vi "Sample Panel2.vi"(8 "error in (no error)":errorcluster, 9 "Left Or Right":string, 10 "Measure_No":i64, 11 "connection reference":T1) -> (0 "error out":errorcluster)   [LabVIEW 2015, in "Sample.lvlib"]
uses:
  Sample.lvlib
  <vilib>/addons/database/Connection.llb/Conn ObjectReference.ctl
  <vilib>/userdefined/High Color/IMAQdx.ctl
  Sub VIs/CCD/CCD.lvlib
  Sub VIs/DAQ/DAQ.lvlib
  <vilib>/vision/driver/NI_Vision_Acquisition_Software.lvlib
  Sub VIs/Digital Signal Processing/Digital Signal Processing.lvlib
  Sub VIs/Utility VIs/Utility VIs.lvlib
  Sub VIs/Database Processing/Database Processing.lvlib
  <vilib>/addons/database/NI_Database_API.lvlib
panel:
  in  "x":bool
  out "Asan Signal":dbl[](graph)
  out "CH1":dbl[](array[numeric])
  in  "停止":bool
  out "CCD Image":T2(plugin-control)
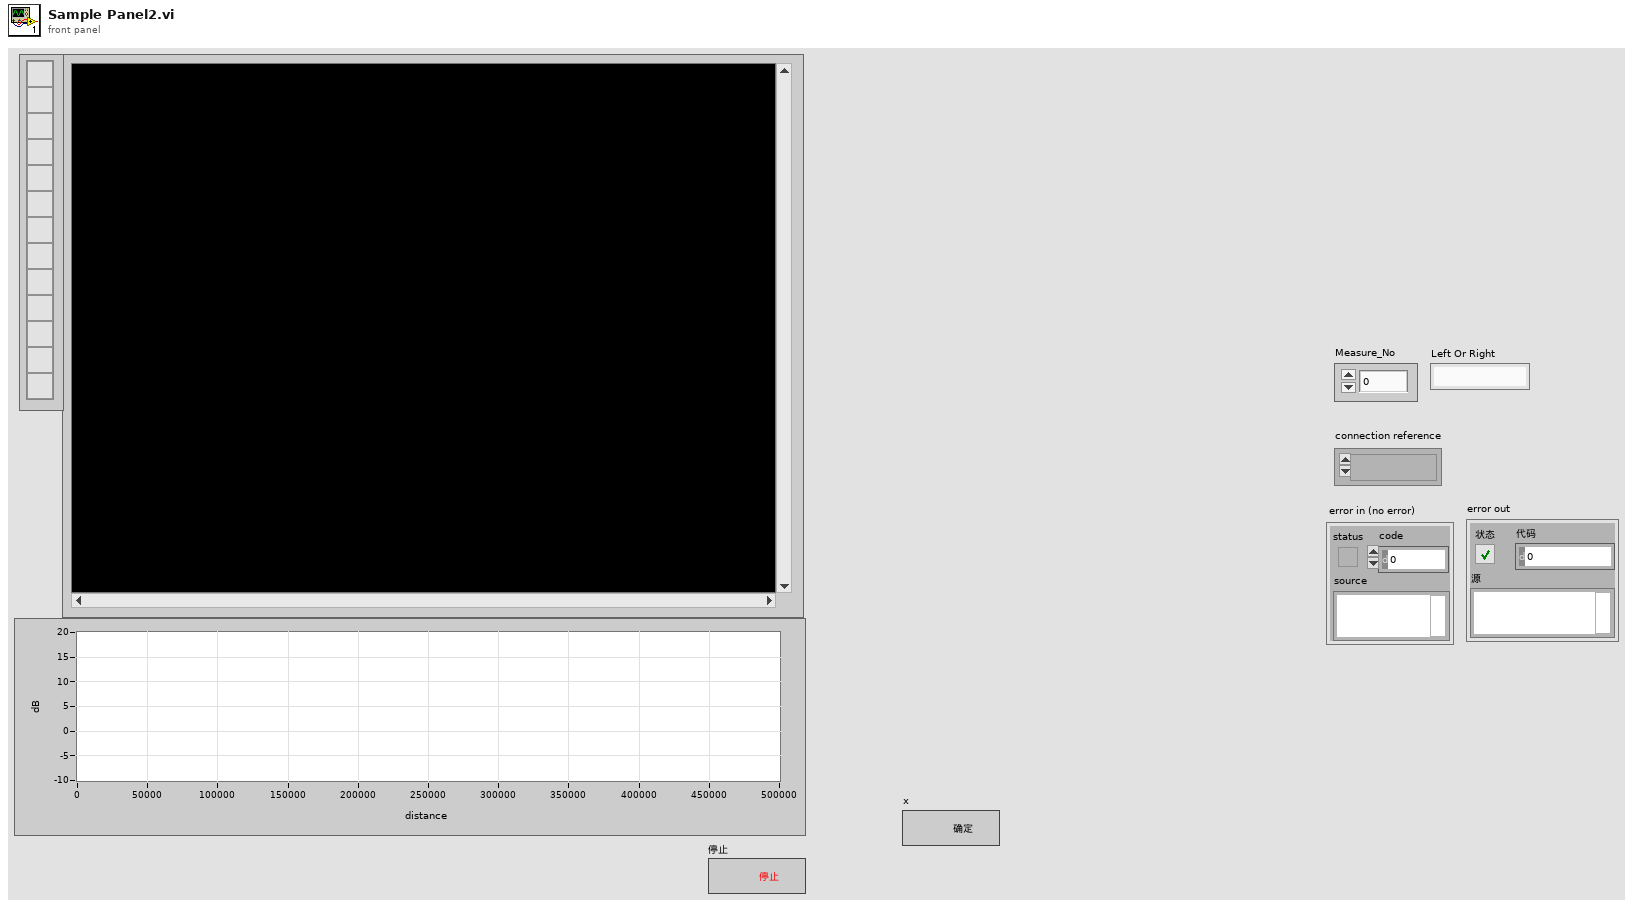
[diagram p1: front panel]
types:
  T1 = typedef "NI_Database_API.lvlib/Conn ObjectReference.ctl" = refnum<k1>
  T2 = typedef "IMAQ Image.ctl" = refnum<image>
  T3 = typedef "IMAQdx.ctl" = refnum<k21>
  T4 = typedef "Database Processing.lvlib/Biometry Attribute.ctl" = cluster{"Measure_ID":i64, "Measure_No":i64, "Ordinal":i64, "L_Or_R":string}
  T5 = typedef "DAQ.lvlib/DAQ Configuration.ctl" = cluster{"hDevice":i32, "DevNum":u8, "Configuration Parameter":i32[], "READ_MAX_LEN":i32, "DO":bool[]}
  T6 = typedef "Digital Signal Processing.lvlib/DSP Configuration.ctl" = cluster{"Sampling Frequency":dbl, "filter type":T7, "RF Filter Low Frequency":dbl, "RF Filter High Frequency":dbl, "RF Filter Taps":i32, "window":T8, "RF window parameter":dbl, "filter type 2":T7, "Demodulated Filter Low Frequency":dbl, "Demodulated Filter HighFrequency":dbl, "Demodulated Filter Order":i32, "SPAN":i32, "Logarithmic Base":dbl, "Noise path":string, "Work position parameter":i32[]}
  T7 = typedef "NI_AALBase.lvlib/Filter Passband Type.ctl" = enum32{"Lowpass", "Highpass", "Bandpass", "Bandstop"}
  T8 = typedef "NI_AALPro.lvlib/windowTd.ctl" = u32
  T9 = typedef "Digital Signal Processing.lvlib/DSP Parameter.ctl" = cluster{"RF":cluster{"filter structure":enum32{"IIR 2nd Order", "IIR 4th Order"}, "Reverse Coefficients":dbl[], "Forward Coefficients":dbl[]}, "IIR Filter Cluster":cluster{"filter structure":enum32{"IIR 2nd Order", "IIR 4th Order"}, "Reverse Coefficients":dbl[], "Forward Coefficients":dbl[]}, "Noise Signal":dbl[], "SPAN":i32, "Logarithmic Base":dbl}
  T10 = cluster{"Measure_ID":i32, "Original Ascan Path":string, "Original IR Path":string, "Original WTW Path":string, "Processing Ascan Path":string, "Processing IR Path":string, "Processing WTW Path":string, "Processing K Path":string, "Processing A Path":string}
  T11 = cluster{"Measure_ID":i32, "Measure_No":i32, "Ordinal":i32, "Left Or Right":string}
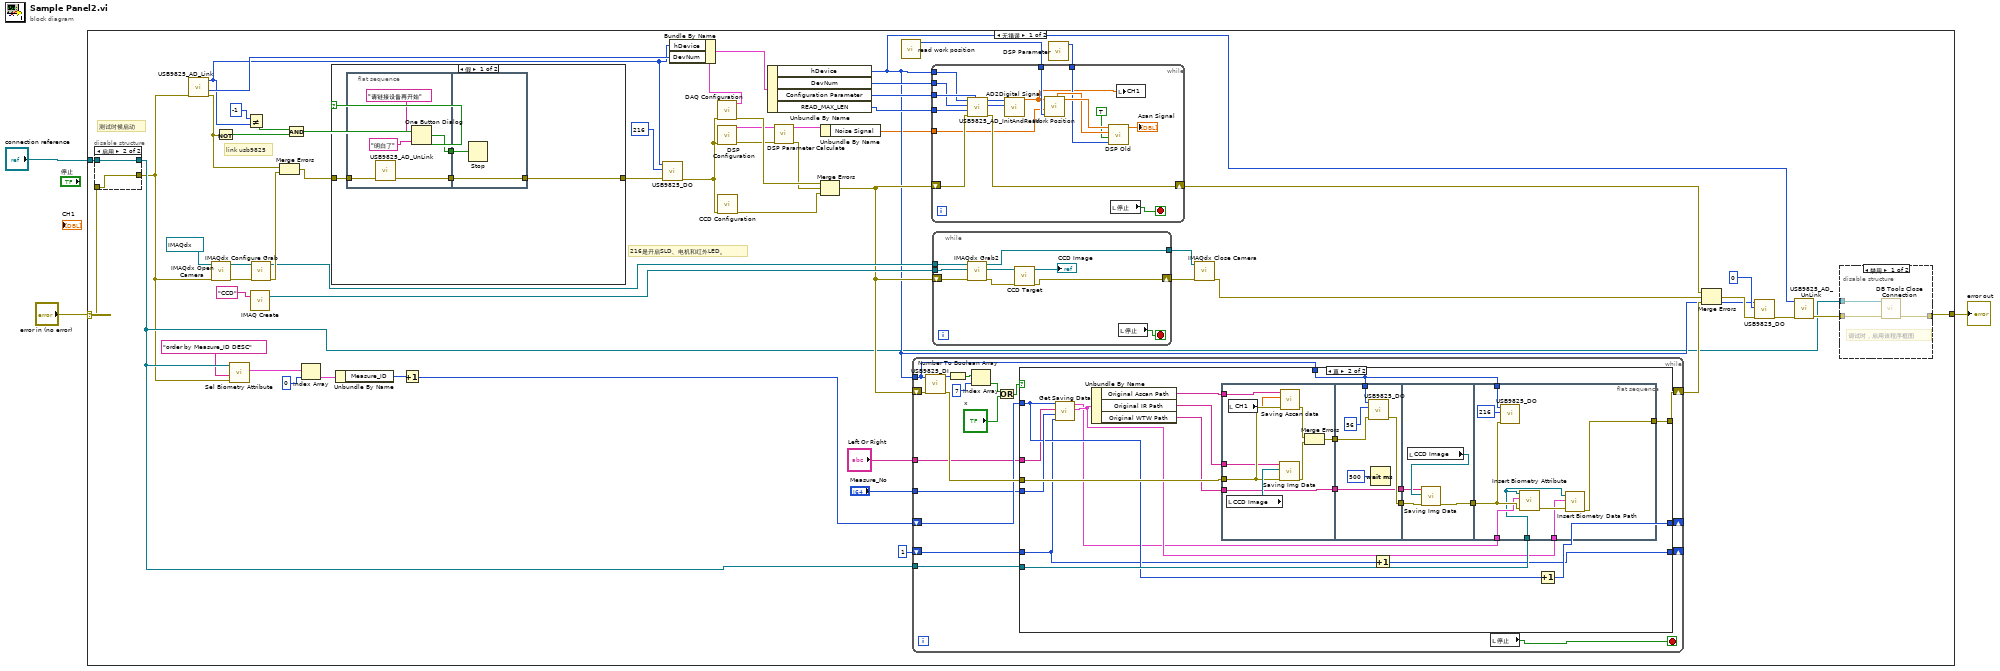
[diagram p0: block diagram]
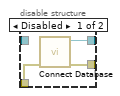
[diagram p3: hidden frame]
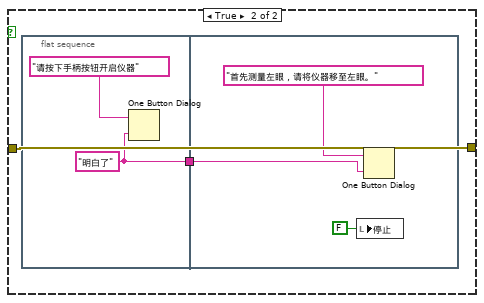
[diagram p5: hidden frame]
diagram:
  n1 = case shown="无错误" "error in (no error)" {
    selector: "error in (no error)" -> [w28 w182]
    tunnel: "connection reference" -> [w27 _]
    tunnel: [w20 w182] -> w1
    frame No Error {
      # "测试时候启动"
      # "216是开启SLD、电机和红外LED。"
      # "link usb9825"
      n2 = disable-structure shown="启用" {
        disable-tunnel: [w67 w68] -> w6
        disable-tunnel: w28 -> [w66 w68]
        disable-tunnel: [w65 w69] -> w8
        disable-tunnel: w27 -> [_ w69]
        frame Disabled {
          n3 = call "Connect Database.vi"("error in (no error)"=w66) -> ("error out"=w67:errorcluster, "connection reference"=w65:T1)  [unwired: 9 in]
        }
        frame Enabled {
        }
      }
      n4 = call "USB9825_AD_Link.vi"("Error In"=w6) -> ("Error Out"=w60:errorcluster, "DevNum"=w34:i32, "hDevice"=w33:i32)  [unwired: 7 in, 1 out]
      n5 = call <vilib>:"IMAQdx Open Camera.vi"("error in"=w6, "Session In"=T3 "cam0") -> ("error out"=w55:errorcluster, "Session Out"=w56:T3)  [unwired: 8 in]
      n6 = Not(x=w60) -> (.not. x?=w51:bool)
      n7 = call "Sel Biometry Attribute.vi"("error in (no error)"=w6, "condition"="order by Measure_ID DESC", "connection reference"=w8) -> ("Biometry Attribute"=w9:T4[])  [unwired: 7 in, 1 out]
      n8 = Not Equal?(x=-1, y=w33) -> (x != y?=w52:bool)
      n9 = call "IMAQ Create"("Image Name"="CCD") -> ("New Image"=w39:T2)  [unwired: 4 in, 1 out]
      n10 = call <vilib>:"IMAQdx Configure Grab.vi"("error in"=w55, "Session In"=w56) -> ("error out"=w53:errorcluster, "Session Out"=w40:T3)  [unwired: 8 in]
      n11 = Merge Errors(w60, w53) -> (w58:errorcluster)
      n12 = And(x=w52, y=w51) -> (x .and. y?=w50:bool)
      n13 = Index Array(array=w9, index=0 ("索引")) -> (element=w26:T4)
      n14 = case shown="假" w50 {
        tunnel: [w167 w175] -> w49
        tunnel: w58 -> [w166 w175]
        frame False {
          n15 = flat-sequence {
            tunnel: [w168] -> w165
            tunnel: w166 -> [w169]
            tunnel: [w170] -> w164
            tunnel: [w173] -> w167
            tunnel: w165 -> [w173]
            tunnel: w164 -> [w174]
            frame #0 {
              n16 = call "USB9825_AD_UnLink.vi"("Error In"=w169) -> ("Error Out"=w168:errorcluster)  [unwired: 10 in]
              n17 = One Button Dialog(message="请链接设备再开始" ("消息"), button name ("OK")="明白了" ("按钮名称（“确定”）")) -> (true=w170:bool)
            }
            frame #1 {
              n18 = Stop(stop? (T)=w174) -> ()
            }
          }
        }
        frame True {
          n19 = flat-sequence {
            tunnel: [w177] -> w176
            tunnel: w176 -> [w181]
            frame #0 {
              w177 = "明白了" ("按钮名称（“确定”）")
              n20 = One Button Dialog(message="请按下手柄按钮开启仪器" ("消息"), button name ("OK")=w177) -> ()  [unwired: 1 out]
            }
            frame #1 {
              n21 = local write "停止"(FALSE ("停止")) -> ()
              n22 = One Button Dialog(message="首先测量左眼，请将仪器移至左眼。" ("消息"), button name ("OK")=w181) -> ()  [unwired: 1 out]
            }
          }
        }
      }
      n23 = Unbundle By Name(w26) -> ("Measure_ID"=w24:i64)
      n24 = Increment(x=w24) -> (x+1=w23:i64)
      n25 = call "USB9825_DO.vi"("Error In"=w49, "pDO"=u8 216, "hDevice"=w33) -> ("Error Out"=w38:errorcluster)  [unwired: 8 in]
      n26 = call "DAQ Configuration.vi"("error in (no error)"=w38) -> ("error out"=w47:errorcluster, "parameter output"=w36:T5)  [unwired: 9 in]
      n27 = Bundle By Name(cluster=w36, "hDevice"=w33, "DevNum"=w34) -> (w35:T5)
      n28 = call "DSP Configuration.vi"("error in (no error)"=w38) -> ("error out"=w44:errorcluster, "DSP Parameter Output"=w46:T6)  [unwired: 9 in]
      n29 = call "CCD Configuration.vi"("error in (no error)"=w38) -> ("error out"=w37:errorcluster)  [unwired: 9 in, 1 out]
      n30 = Unbundle By Name(w35) -> ("hDevice"=w14:i32, "DevNum"=w42:u8, "Configuration Parameter"=w43:i32[], "READ_MAX_LEN"=w41:i32)
      n31 = call "DSP Parameter Calculate.vi"("error in (no error)"=w44, "DSP Configuration"=w46) -> ("error out"=w45:errorcluster, "DSP Parameter"=w5:T9)  [unwired: 8 in]
      n32 = Unbundle By Name(w5) -> ("Noise Signal"=w4:dbl[])
      n33 = Merge Errors(w47, w45, w37) -> (w32:errorcluster)
      n34 = call "read work position.vi"() -> ("Work Position"=w19:i32[])  [unwired: 10 in, 1 out]
      n35 = while {
        tunnel: w14 -> [w82]
        shift-right: [w81] -> w30
        shift-left: w32 -> [w87]
        shift-right: [w80] -> _
        shift-left: i64 1 -> [w78]
        tunnel: w8 -> [w75]
        tunnel: "Measure_No" -> [w76]
        shift-right: [w74] -> _
        shift-left: w23 -> [w79]
        tunnel: "Left Or Right" -> [w70]
        stop <- w77 stop-if-true
        n36 = call "USB9825_DI.vi"("错误输入（无错误）"=w87, "hDevice"=w82) -> ("错误输出"=w83:errorcluster, "pDI"=w84:u8)  [unwired: 8 in]
        n37 = Number To Boolean Array(number=w84) -> (Boolean array=w86:bool[])
        n38 = Index Array(array=w86, index=7 ("索引")) -> (element=w72:bool)
        n39 = Or(x=w72, y="x") -> (x .or. y?=w73:bool)
        n40 = case shown="真" w73 {
          tunnel: w83 -> [w89 w110]
          tunnel: w82 -> [_ w106]
          tunnel: [w89 w91] -> w81
          tunnel: [w90 w95] -> w80
          tunnel: w78 -> [w90 w96]
          tunnel: w79 -> [w88 w97]
          tunnel: w76 -> [_ w100]
          tunnel: w75 -> [_ w99]
          tunnel: [w88 w98] -> w74
          tunnel: w70 -> [_ w94]
          frame False {
          }
          frame True {
            n41 = call "Get Saving Data.vi"("Ordinal"=w96, "Measure_No"=w100, "Left Or Right"=w94, "Measure_ID"=w97) -> ("Get Saving Data Path"=w93:T10, "Biometry Attribute"=w92:T11)  [unwired: 6 in]
            n42 = Unbundle By Name(w93) -> ("Original Ascan Path"=w105:string, "Original IR Path"=w104:string, "Original WTW Path"=w101:string)
            n43 = flat-sequence {
              tunnel: w110 -> [w118]
              tunnel: [w115] -> w109
              tunnel: w105 -> [w114]
              tunnel: w104 -> [w113]
              tunnel: [w112] -> w102
              tunnel: w101 -> [w112]
              tunnel: w109 -> [w124]
              tunnel: w106 -> [w123]
              tunnel: [w121] -> w108
              tunnel: [w120] -> w103
              tunnel: w102 -> [w120]
              tunnel: w108 -> [w129]
              tunnel: [w127] -> w107
              tunnel: w103 -> [w126]
              tunnel: w107 -> [w135]
              tunnel: w106 -> [w137]
              tunnel: w99 -> [w133]
              tunnel: w93 -> [w131]
              tunnel: w92 -> [w134]
              tunnel: [w130] -> w91
              frame #0 {
                n44 = local read "CCD Image"() -> (w119:T2)
                n45 = local read "CH1"() -> (w111:dbl[])
                n46 = call "Saving Img Data.vi"("error in (no error)"=w118, "Image"=w119, "名称或相对路径"=w113) -> ("error out"=w117:errorcluster)  [unwired: 8 in]
                n47 = call "Saving Ascan data.vi"("error in (no error)"=w118, "Ascan Data"=w111, "名称或相对路径"=w114) -> ("error out"=w116:errorcluster)  [unwired: 8 in]
                n48 = Merge Errors(w116, w117) -> (w115:errorcluster)
              }
              frame #1 {
                n49 = call "USB9825_DO.vi"("Error In"=w124, "pDO"=u8 56, "hDevice"=w123) -> ("Error Out"=w121:errorcluster)  [unwired: 8 in]
                n50 = Wait (ms)(milliseconds to wait=u32 500 ("等待时间（毫秒）")) -> ()  [unwired: 1 out]
              }
              frame #2 {
                n51 = local read "CCD Image"() -> (w128:T2)
                n52 = call "Saving Img Data.vi"("error in (no error)"=w129, "Image"=w128, "名称或相对路径"=w126) -> ("error out"=w127:errorcluster)  [unwired: 8 in]
              }
              frame #3 {
                n53 = call "USB9825_DO.vi"("Error In"=w135, "pDO"=u8 216, "hDevice"=w137) -> ()  [unwired: 8 in, 1 out]
                n54 = call "Insert Biometry Attribute.vi"("error in (no error)"=w135, "Biometry Attribute Input"=w134, "connection reference"=w133) -> ("error out"=w132:errorcluster)  [unwired: 8 in]
                n55 = call "Insert Biometry Data Path.vi"("error in (no error)"=w132, "Biometry Data Path"=w131, "connection reference"=w133) -> ("error out"=w130:errorcluster)  [unwired: 8 in]
              }
            }
            n56 = Increment(x=w96) -> (x+1=w95:i64)
            n57 = Increment(x=w97) -> (x+1=w98:i64)
          }
        }
        n58 = local read "停止"() -> (w77:bool)
      }
      n59 = while {
        tunnel: w40 -> [w146]
        tunnel: w39 -> [w145]
        shift-right: [w140] -> w17
        shift-left: w32 -> [w144]
        tunnel: [w138] -> w16
        stop <- w139 stop-if-true
        n60 = call <vilib>:"IMAQdx Grab2.vi"("error in"=w144, "Image In"=w145, "Session In"=w146) -> ("error out"=w142:errorcluster, "Image Out"=w143:T2, "Session Out"=w138:T3)  [unwired: 5 in, 1 out]
        n61 = call "CCD Target.vi"("error in (no error)"=w142, "Image"=w143) -> ("error out"=w140:errorcluster, "Image Out"=→"CCD Image":T2)  [unwired: 8 in]
        n62 = local read "停止"() -> (w139:bool)
      }
      n63 = call "DSP Parameter.vi"() -> ("DSP Parameter"=w18:i32[])  [unwired: 10 in, 1 out]
      n64 = while {
        tunnel: w43 -> [w163]
        tunnel: w14 -> [w162]
        tunnel: w42 -> [w161]
        tunnel: w41 -> [w160]
        shift-right: [w149] -> w13
        shift-left: w32 -> [w159]
        tunnel: w19 -> [w155]
        tunnel: w18 -> [w151]
        tunnel: w4 -> [w147]
        stop <- w156 stop-if-true
        n65 = call "USB9825_AD_InitAndRead.vi"("Configuration Parameter"=w163, "错误输入（无错误）"=w159, "READ_MAX_LEN"=w160, "DevNum"=w161, "hDevice"=w162) -> ("错误输出"=w149:errorcluster, "通道数"=w157:i32, "AD"=w158:i16[])  [unwired: 4 in]
        n66 = call "AD2Digital Signal.vi"("通道数"=w157, "AD"=w158) -> ("CH1"=w148:dbl[])  [unwired: 8 in, 1 out]
        n67 = call "Work Position.vi"("Work position parameter"=w155, "Noise"=w147, "S"=w148) -> ("S_1st_part"=w154:dbl[], "Noise_1st_part"=w153:dbl[])  [unwired: 3 in, 4 out]
        n68 = call "DSP Old.vi"("DSP Parameter"=w151, "Minus Noise(F : Don't)"=TRUE, "Noise Signal"=w153, "Input Signal"=w154) -> ("DSP signal"=→"Asan Signal":dbl[])  [unwired: 7 in]
        n69 = local read "停止"() -> (w156:bool)
        n70 = local write "CH1"(w148) -> ()
      }
      n71 = call <vilib>:"IMAQdx Close Camera.vi"("error in"=w17, "Session In"=w16) -> ("error out"=w15:errorcluster)  [unwired: 9 in]
      n72 = Merge Errors(w13, w15, w30) -> (w29:errorcluster)
      n73 = call "USB9825_DO.vi"("Error In"=w29, "pDO"=u8 0, "hDevice"=w14) -> ("Error Out"=w12:errorcluster)  [unwired: 8 in]
      n74 = call "USB9825_AD_UnLink.vi"("Error In"=w12, "hDevice"=w14) -> ("Error Out"=w11:errorcluster)  [unwired: 9 in]
      n75 = disable-structure shown="禁用" {
        disable-tunnel: w8 -> [w63 _]
        disable-tunnel: w11 -> [w62 w64]
        disable-tunnel: [w61 w64] -> w20
        frame Disabled {
          # "调试时，启用该程序框图"
          n76 = call <vilib>:"DB Tools Close Connection.vi"("error in (no error)"=w62, "connection reference"=w63) -> ("error out"=w61:errorcluster)  [unwired: 5 in]
        }
        frame Enabled {
        }
      }
    }
    frame Error {
    }
  }
  "error out" <- w1
